vi "1D upper limit bounce.vi"(7 "starting state":T1={"position (m)"=5.0, "velocity (m/s)"=10.0}, 11 "coefficient of restitution [0.9]":dbl=0.9 min=0.0 max=1.0 step=0.001, 13 "upper limit (m)":dbl=10.0 min=0.0 max=1.0 step=0.001) -> (8 "ending state":T1={"position (m)"=5.0, "velocity (m/s)"=10.0})   [LabVIEW 2016]
doc: "This subvi updates the velocity and position of an object due to a bounce off an upper wall given the coefficient of restitution.\n\nPaul K Dixon\nP350\nCSUSB Physics"
uses:
  typedef/1d state.ctl
panel:
  # "Upper Limit"
  # "update parameters"
  # "Paul K Dixon\nP350"
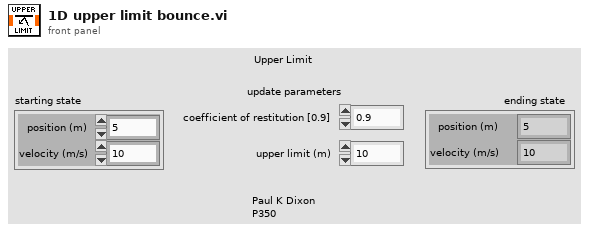
[diagram p1: front panel]
types:
  T1 = typedef "1d state.ctl" = cluster{"position (m)":dbl, "velocity (m/s)":dbl}
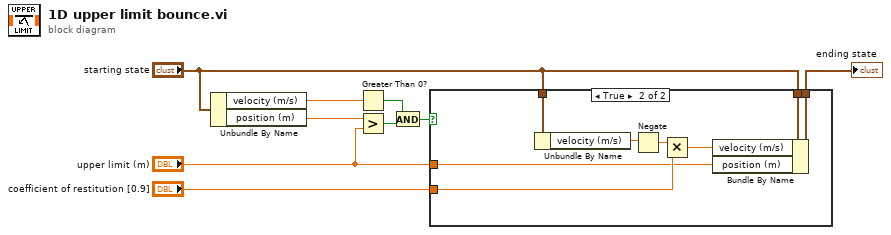
[diagram p0: block diagram]
diagram:
  n1 = Unbundle By Name("starting state") -> ("velocity (m/s)"=w8:dbl, "position (m)"=w3:dbl)
  n2 = Greater Than 0?(x=w8) -> (x > 0?=w6:bool)
  n3 = Greater?(x=w3, y="upper limit (m)") -> (0:w2:bool)
  n4 = And(x=w6, y=w2) -> (x .and. y?=w7:bool)
  n5 = case shown="True" w7 {
    tunnel: "starting state" -> [w10 w18]
    tunnel: [w10 w17] -> w9
    tunnel: "starting state" -> [_ w16]
    tunnel: "coefficient of restitution [0.9]" -> [_ w13]
    tunnel: "upper limit (m)" -> [_ w11]
    frame False {
    }
    frame True {
      n6 = Unbundle By Name(w16) -> ("velocity (m/s)"=w15:dbl)
      n7 = Negate(x=w15) -> (-x=w14:dbl)
      n8 = Multiply(x=w14, y=w13) -> (x*y=w12:dbl)
      n9 = Bundle By Name(cluster=w18, "velocity (m/s)"=w12, "position (m)"=w11) -> (w17:T1)
    }
  }
  "ending state" <- w9
